vi "Render.vi"(8 "error in":errorcluster, 10 "Renderer in":refnum<class "Renderer.lvclass">, 11 "Classes Overview in":refnum<class "Classes Overview.lvclass">) -> (0 "error out":errorcluster, 3 "Sections out":refnum<class "Section.lvclass">[](array[class]))   [LabVIEW 2021, in "TAF Proj Document Type.lvlib" / "Classes Overview.lvclass"]
uses:
  <vilib>/Wovalab/AntiDoc/Document Type/Add-ons/LabVIEW TAF Project/Classes Overview/Classes Overview.lvclass
  C:/Program Files (x86)/National Instruments/LabVIEW 2021/vi.lib/Wovalab/AntiDoc/Bloc/Bloc.lvclass
  <vilib>/Wovalab/AsciiDoc for LabVIEW/Section/Section.lvclass
  <vilib>/Wovalab/AntiDoc/Renderer/Renderer.lvclass
  <vilib>/Wovalab/AsciiDoc for LabVIEW/Diagram/Type--enum.ctl
  <vilib>/Wovalab/AntiDoc/Document Type/Add-ons/LabVIEW TAF Project/Classes Overview/Classes Overview.lvclass/Classes Overview.ctl
  <vilib>/Wovalab/AntiDoc/Bloc/Bloc.lvclass/Bloc.ctl
  <vilib>/Wovalab/AntiDoc/Document Type/Add-ons/LabVIEW TAF Project/Class/Class.lvclass/Class.ctl
  <vilib>/Wovalab/AsciiDoc for LabVIEW/Table/Table.lvclass/Table.ctl
  <vilib>/Wovalab/AntiDoc/Bloc/Read Name.vi
  <vilib>/Wovalab/AntiDoc/Document Type/Add-ons/LabVIEW TAF Project/Class/Read Is Interface.vi
  <vilib>/Wovalab/AntiDoc/Document Type/Add-ons/LabVIEW TAF Project/Class/Class.lvclass
  <vilib>/Wovalab/AsciiDoc for LabVIEW/Paragraph/Paragraph.lvclass
  C:/Program Files (x86)/National Instruments/LabVIEW 2021/vi.lib/Wovalab/AsciiDoc for LabVIEW/Adoc-Bloc/Bloc.lvclass
  <vilib>/Wovalab/AsciiDoc for LabVIEW/Table/Table.lvclass
  <vilib>/Wovalab/AsciiDoc for LabVIEW/Diagram/Diagram.lvclass
  <vilib>/Wovalab/AsciiDoc for LabVIEW/Section/Add Bloc (array).vi
  <vilib>/Wovalab/AntiDoc/Document Type/Add-ons/LabVIEW TAF Project/TAF Proj Document Type.lvlib
  <vilib>/Wovalab/AntiDoc/Utilities/Utilities.lvlib
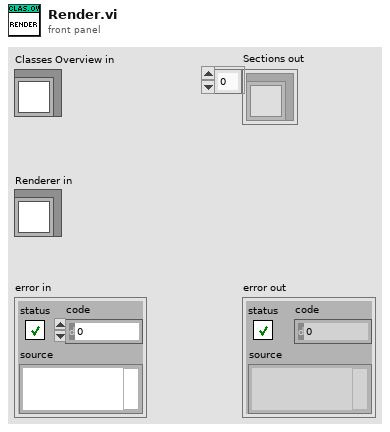
[diagram p1: front panel]
types:
  T1 = typedef "Wovalab_lib_AsciiDoctor.lvlib/Diagram.lvclass/Type--enum.ctl" = enum16{"a2s", "actdiag", "blockdiag", "ditaa", "erd", "graphviz", "meme", "mermaid", "msc", "nwdiag", "packetdiag", "plantuml", "rackdiag", "seqdiag", "shaape", "svgbob", "syntrax", "umlet", "vega", "vegalite", "wavedrom"}
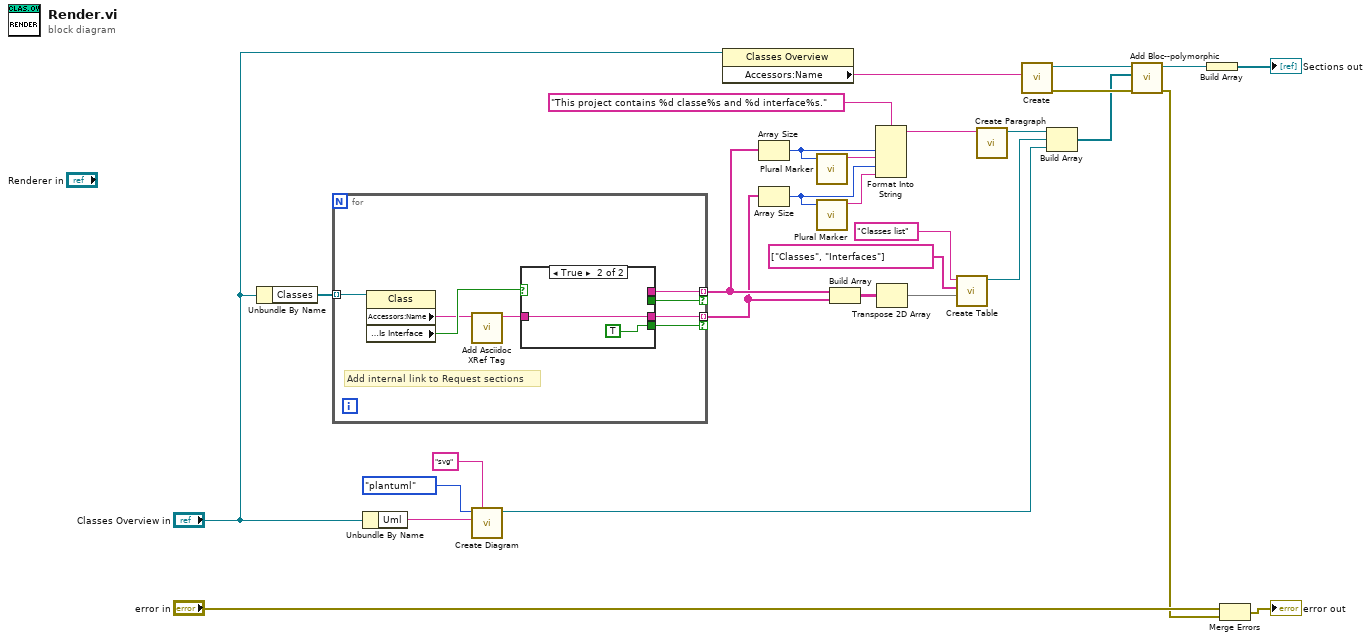
[diagram p0: block diagram]
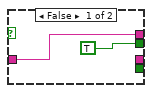
[diagram p2: hidden frame]
diagram:
  n1 = Unbundle By Name("Classes Overview in") -> ("Classes"=w16:refnum<class "Class.lvclass">[])
  n2 = for {
    tunnel: w16 -> [w37] mode=indexing
    tunnel: [w35] -> w12 mode=indexing if=w33
    tunnel: [w34] -> w9 mode=indexing if=w32
    # "Add internal link to Request sections"
    n3 = property class="Class"(reference=w37) -> ("Accessors:Name"=w31:string, "Accessors:Is Interface"=w36:bool)  [unwired: 1 in, 2 out]
    n4 = call <vilib>:"Add Asciidoc XRef Tag.vi"("String In"=w31) -> ("String out"=w30:string)  [unwired: 10 in]
    n5 = case shown="True" w36 {
      tunnel: [_ w41] -> w34
      tunnel: w30 -> [w39 w41]
      tunnel: [w39 _] -> w35
      tunnel: [_ TRUE] -> w32
      tunnel: [TRUE _] -> w33
      frame False {
      }
      frame True {
      }
    }
  }
  n6 = Unbundle By Name("Classes Overview in") -> ("Uml"=w24:string)
  n7 = call <vilib>:"Create Diagram.vi"("Format (png)"="svg", "Diagram Source Code"=w24, "Diagram Type"=Type--enum."plantuml") -> ("Diagram out"=w22:refnum<class "Diagram.lvclass">)  [unwired: 7 in, 1 out]
  n8 = property class="Classes Overview"(reference="Classes Overview in") -> ("Accessors:Name"=w3:string)  [unwired: 1 in, 2 out]
  n9 = Array Size(array=w12) -> (size(s)=w8:i32)
  n10 = Array Size(array=w9) -> (size(s)=w6:i32)
  n11 = call <vilib>:"Plural Marker.vi"("Size"=w8) -> ("Plural Mark"=w7:string)  [unwired: 10 in]
  n12 = call <vilib>:"Plural Marker.vi"("Size"=w6) -> ("Plural Mark"=w5:string)  [unwired: 10 in]
  n13 = Build Array(w12, w9) -> (w18:string[][])
  n14 = Format Into String(format string="This project contains %d classe%s and %d interface%s." ("Content"), w8, w7, w6, w5) -> (resulting string=w11:string)  [unwired: 2 in, 1 out]
  n15 = Transpose 2D Array(2D array=w18) -> (transposed array=w17:string[][])
  n16 = call <vilib>:"Create Table.vi"("Content"=w17, "Header"=string[] ["Classes", "Interfaces"], "Title"="Classes list") -> ("Table out"=w14:refnum<class "Table.lvclass">)  [unwired: 7 in, 1 out]
  n17 = call <vilib>:"Create Paragraph.vi"("Content"=w11) -> ("Paragraph out"=w13:refnum<class "Paragraph.lvclass">)  [unwired: 9 in, 1 out]
  n18 = call <vilib>:"Create.vi"("Title"=w3) -> ("error out"=w29:errorcluster, "Section out"=w25:refnum<class "Section.lvclass">)  [unwired: 9 in]
  n19 = Build Array(w13, w14, w22) -> (w15:refnum<class "Bloc.lvclass">[])
  n20 = call-poly <vilib>:"Add Bloc--polymorphic.vi"("error in"=w29, "Bloc"=w15, "Section in"=w25) -> ("error out"=w26:errorcluster, "Section out"=w2:refnum<class "Section.lvclass">)  [unwired: 7 in]
  n21 = Build Array(w2) -> (→"Sections out":refnum<class "Section.lvclass">[])
  n22 = Merge Errors("error in", w26) -> (→"error out":errorcluster)
